vi "4461 Autophase.vi"(8 "error in (no error)":errorcluster, 10 "Results":T1, 11 "LockinDAQ":refnum<class "LockinDAQ.lvclass">) -> (0 "error out":errorcluster, 3 "LockinDAQ out":refnum<class "LockinDAQ.lvclass">)   [LabVIEW 2016, in "LockinDAQ.lvclass"]
uses:
  LockinDAQ.lvclass
  Typedefs/Results--Cluster.ctl
  LockinDAQ.lvclass/LockinDAQ.ctl
panel:
  in  "D":dbl=0.019999999999999997 format="%.2f"
  in  "I":dbl=0.6 format="%.2f"
  in  "P":dbl=0.5 format="%.2f"
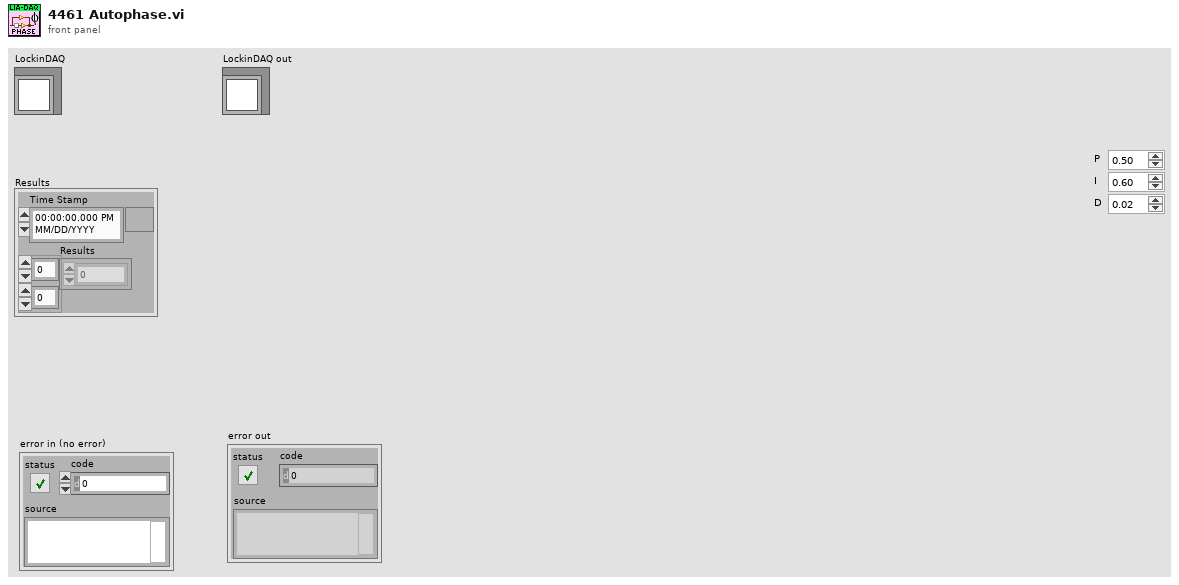
[diagram p1: front panel]
types:
  T1 = typedef "LockinDAQ.lvclass/Results--Cluster.ctl" = cluster{"Time Stamp":timestamp, "Results":dbl[][]}
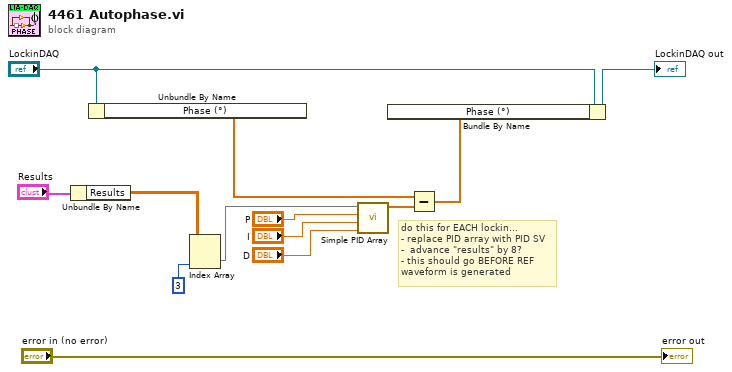
[diagram p0: block diagram]
diagram:
  # "do this for EACH lockin...\n- replace PID array with PID SV\n-  advance \"results\" by 8?\n- this should go BEFORE REF\nwaveform is generated"
  n1 = Unbundle By Name("Results") -> ("Results"=w1:dbl[][])
  n2 = Unbundle By Name("LockinDAQ") -> ("Phase (°)"=w3:dbl[])
  n3 = Index Array(array=w1, index (col)=3 ("index (row)")) -> (element=w8:dbl[])  [unwired: 1 in]
  n4 = call "Simple PID Array.vi"("D"="D", "I"="I", "P"="P", "process variable"=w8) -> ("output value"=w12:dbl[])  [unwired: 7 in]
  n5 = Subtract(x=w3, y=w12) -> (x-y=w6:dbl[])
  n6 = Bundle By Name(cluster="LockinDAQ", "Phase (°)"=w6) -> (→"LockinDAQ out":refnum<class "LockinDAQ.lvclass">)
  "error out" <- "error in (no error)"
